vi "Speckle variance OCTA.vi"() -> ()   [LabVIEW 2018]
uses:
  <vilib>/ptbypt/NI_PtbyPt.lvlib
panel:
  in  "#SPK":i32
  in  "# Bscan":i32=400
  in  "Array":sgl[][][][](array[numeric])
  in  "# Ascan":i32=400
  in  "Z length (pix)":i32=1024
  out "?":dbl[][](graph)
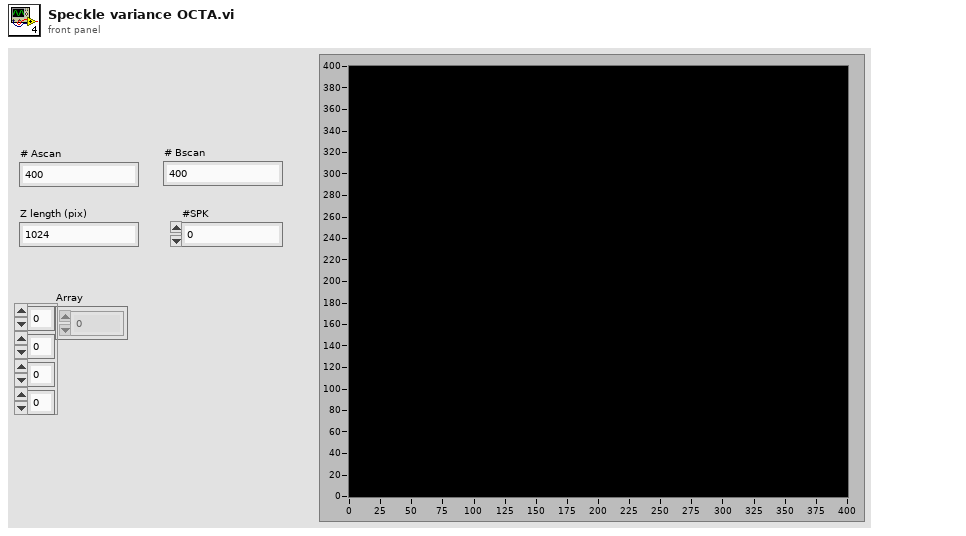
[diagram p1: front panel]
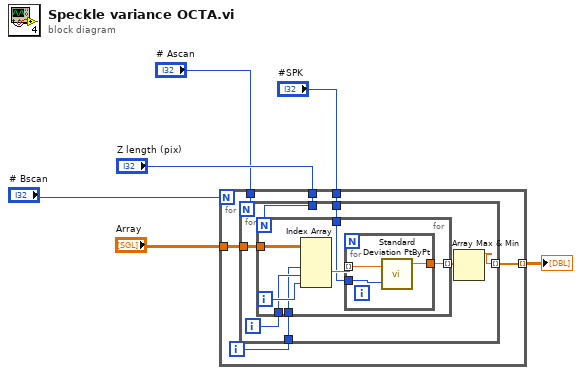
[diagram p0: block diagram]
diagram:
  n1 = for {
    N: "# Bscan" -> [_]
    tunnel: "Array" -> [w12]
    tunnel: "#SPK" -> [w10]
    tunnel: [w9] -> w6 mode=indexing
    tunnel: "Z length (pix)" -> [w8]
    tunnel: "# Ascan" -> [w7]
    i -> [w11]
    n2 = for {
      N: w7 -> [_]
      tunnel: w12 -> [w19]
      tunnel: w11 -> [w17]
      tunnel: w10 -> [w16]
      tunnel: [w14] -> w9 mode=indexing
      tunnel: w8 -> [w13]
      i -> [w18]
      n3 = for {
        N: w13 -> [_]
        tunnel: w19 -> [w26]
        tunnel: w18 -> [w24]
        tunnel: w17 -> [w23]
        tunnel: w16 -> [w21]
        tunnel: [w20] -> w15 mode=indexing
        i -> [w25]
        n4 = Index Array(array=w26, index (dim 1)=w23, index (dim 2)=w24, index (dim 3)=w25) -> (element=w22:sgl[])  [unwired: 1 in]
        n5 = for {
          tunnel: w22 -> [w29] mode=indexing
          tunnel: w21 -> [w28]
          tunnel: [w27] -> w20
          n6 = call <vilib>:"Standard Deviation PtByPt.vi"("x"=w29, "sample length"=w28) -> ("standard deviation"=w27:dbl)  [unwired: 1 in, 2 out]
        }
      }
      n7 = Array Max & Min(array=w15) -> (max value=w14:dbl)  [unwired: 3 out]
    }
  }
  "?" <- w6
